vi "Handle.vi"(8 "error in (no error)":errorcluster, 11 "TCS in":refnum<class "TCS.lvclass">) -> (0 "error out":errorcluster, 3 "TCS out":refnum<class "TCS.lvclass">)   [LabVIEW 2018, in "TCS.lvclass"]
uses:
  TCS.lvclass
  TCS.lvclass/TCS.ctl
  Device/Device.lvclass/Device.ctl
  Telemetry/Telemetry.lvclass
  C:/Users/observer/Desktop/Sparc4GUI/Versao ZeroMQ/SPARC4_GUI - projeto para EXE - 20240702/Device/Device.lvclass
  Server/Server.lvclass
  Comm/Stream/Stream.lvclass
  Device/Device.lvclass
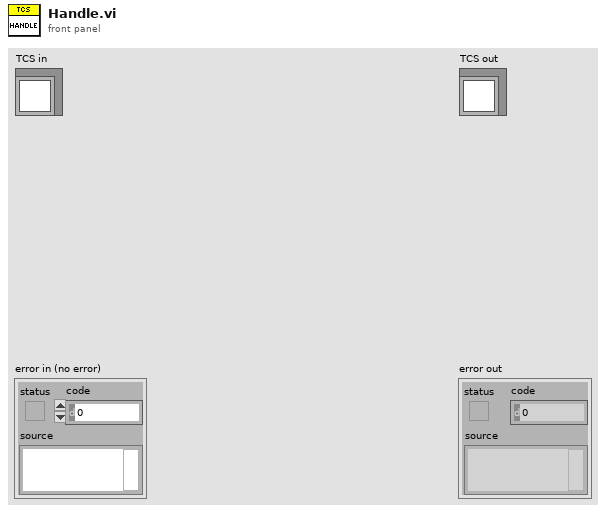
[diagram p1: front panel]
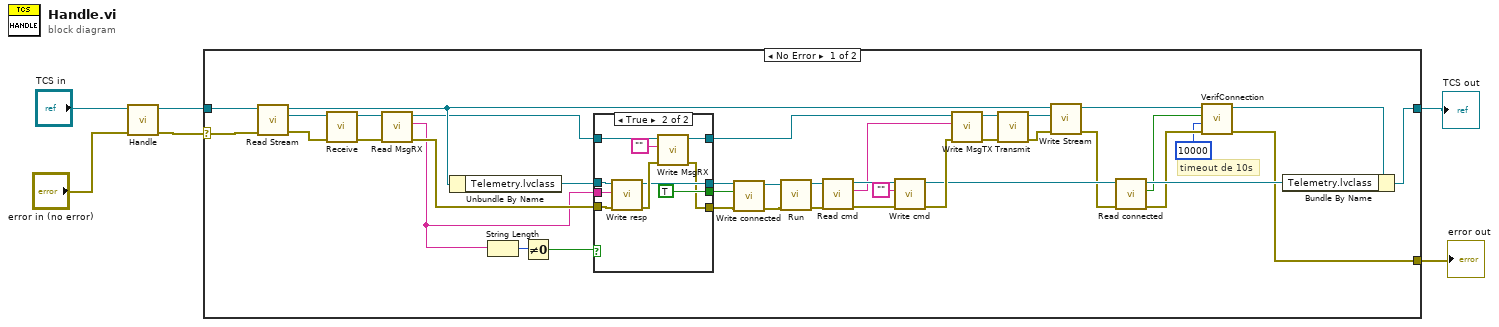
[diagram p0: block diagram]
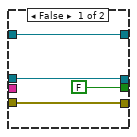
[diagram p2: hidden frame]
diagram:
  n1 = call-parent "Handle.vi"("error in (no error)"="error in (no error)", "Server in"="TCS in") -> ("error out"=w3:errorcluster, "Server out"=w4:refnum<class "TCS.lvclass">)  [unwired: 8 in]
  n2 = case shown="No Error" w3 {
    selector: w3 -> [w44 w62]
    tunnel: [w18 w62] -> w1
    tunnel: [w43 w61] -> w2
    tunnel: w4 -> [w35 w61]
    frame No Error {
      # "timeout de 10s"
      n3 = call-dynamic "Read Stream.vi"("error in (no error)"=w44, "Server in"=w35) -> ("error out"=w45:errorcluster, "Stream.lvclass"=w46:refnum<class "Stream.lvclass">, "Server out"=w37:refnum<class "TCS.lvclass">)  [unwired: 7 in]
      n4 = call-dynamic "Receive.vi"("error in (no error)"=w45, "Stream in"=w46) -> ("error out"=w42:errorcluster, "Stream out"=w41:refnum<class "Stream.lvclass">)  [unwired: 8 in]
      n5 = call-dynamic "Read MsgRX.vi"("error in (no error)"=w42, "Comm in"=w41) -> ("error out"=w8:errorcluster, "MsgRX"=w7:string, "Comm out"=w16:refnum<class "Stream.lvclass">)  [unwired: 7 in]
      n6 = Unbundle By Name(w37) -> ("Telemetry.lvclass"=w9:refnum<class "Telemetry.lvclass">)
      n7 = String Length(string=w7) -> (length=w29:i32)
      n8 = Not Equal To 0?(x=w29) -> (x != 0?=w28:bool)
      n9 = case shown="True" w28 {
        tunnel: [w49 w51] -> w12
        tunnel: [w50 w53] -> w14
        tunnel: w8 -> [w49 w55]
        tunnel: w9 -> [w50 w57]
        tunnel: w16 -> [w48 w60]
        tunnel: [w48 w59] -> w15
        tunnel: [FALSE TRUE] -> w10
        tunnel: w7 -> [_ w54]
        frame False {
        }
        frame True {
          n10 = call-dynamic "Write resp.vi"("error in (no error)"=w55, "resp"=w54, "Device in"=w57) -> ("error out"=w56:errorcluster, "Device out"=w53:refnum<class "Telemetry.lvclass">)  [unwired: 7 in]
          n11 = call-dynamic "Write MsgRX.vi"("error in (no error)"=w56, "MsgRX"="", "Comm in"=w60) -> ("error out"=w51:errorcluster, "Comm out"=w59:refnum<class "Stream.lvclass">)  [unwired: 7 in]
        }
      }
      n12 = call "Write connected.vi"("error in (no error)"=w12, "connected"=w10, "Device in"=w14) -> ("error out"=w11:errorcluster, "Device out"=w13:refnum<class "Telemetry.lvclass">)  [unwired: 7 in]
      n13 = call-dynamic "Run.vi"("error in (no error)"=w11, "Telemetry in"=w13) -> ("error out"=w26:errorcluster, "Telemetry out"=w27:refnum<class "Telemetry.lvclass">)  [unwired: 8 in]
      n14 = call-dynamic "Read cmd.vi"("error in (no error)"=w26, "Device in"=w27) -> ("error out"=w33:errorcluster, "cmd"=w31:string, "Device out"=w34:refnum<class "Telemetry.lvclass">)  [unwired: 7 in]
      n15 = call-dynamic "Write cmd.vi"("error in (no error)"=w33, "cmd"="", "Device in"=w34) -> ("error out"=w40:errorcluster, "Device out"=w25:refnum<class "Telemetry.lvclass">)  [unwired: 7 in]
      n16 = call-dynamic "Write MsgTX.vi"("error in (no error)"=w40, "MsgTX"=w31, "Comm in"=w15) -> ("error out"=w38:errorcluster, "Comm out"=w39:refnum<class "Stream.lvclass">)  [unwired: 7 in]
      n17 = call-dynamic "Transmit.vi"("error in (no error)"=w38, "Stream in"=w39) -> ("error out"=w36:errorcluster, "Stream out"=w30:refnum<class "Stream.lvclass">)  [unwired: 8 in]
      n18 = call-dynamic "Write Stream.vi"("error in (no error)"=w36, "Stream.lvclass"=w30, "Server in"=w37) -> ("error out"=w24:errorcluster, "Server out"=w23:refnum<class "TCS.lvclass">)  [unwired: 7 in]
      n19 = call "Read connected.vi"("error in (no error)"=w24, "Device in"=w25) -> ("error out"=w19:errorcluster, "connected"=w21:bool, "Device out"=w22:refnum<class "Telemetry.lvclass">)  [unwired: 7 in]
      n20 = call-dynamic "VerifConnection.vi"("error in (no error)"=w19, "timeout in ms (1000)"=u32 10000 ("period (ms)"), "device connected in"=w21, "Server in"=w23) -> ("error out"=w18:errorcluster, "Server out"=w20:refnum<class "TCS.lvclass">)  [unwired: 6 in]
      n21 = Bundle By Name(cluster=w20, "Telemetry.lvclass"=w22) -> (w43:refnum<class "TCS.lvclass">)
    }
    frame Error {
    }
  }
  "error out" <- w1
  "TCS out" <- w2
